vi "Merge Error.vi"(10 "Error":errorcluster, 11 "Set Error in":refnum<class "Merge Error.lvclass">) -> (3 "Set Error out":refnum<class "Merge Error.lvclass">)   [LabVIEW 2021, in "Merge Error.lvlib" / "Merge Error.lvclass"]
uses:
  Merge Error.lvclass
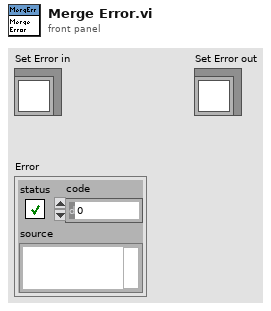
[diagram p1: front panel]
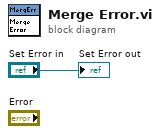
[diagram p0: block diagram]
diagram:
  "Set Error out" <- "Set Error in"
